vi "Change Setting.vi"(7 "Data":string, 8 "error in (no error)":errorcluster, 9 "Device and Axis":string, 10 "Setting":string, 11 "VISA resource name":refnum<visa-resource-name>) -> (0 "error out":errorcluster, 3 "VISA resource name out":refnum<visa-resource-name>)   [LabVIEW 2013, in "Zaber A Series.lvlib"]
doc: "Changes a setting from the device. Omitting the Device and Axis will change the settings of all connected devices. See a list of settings available here: http://www.zaber.com/wiki/Manuals/ASCII_Protocol_Manual#Device_Settings. You do not need to include the 'set' command with this VI, you only need to input the setting you'd like to change. \n\nThe Detect Devices VI is designed to provide an easy list of valid Device and Axis inputs. \n\nThis VI requires that the Initialize VI has been called with the same serial port."
uses:
  Zaber A Series.lvlib
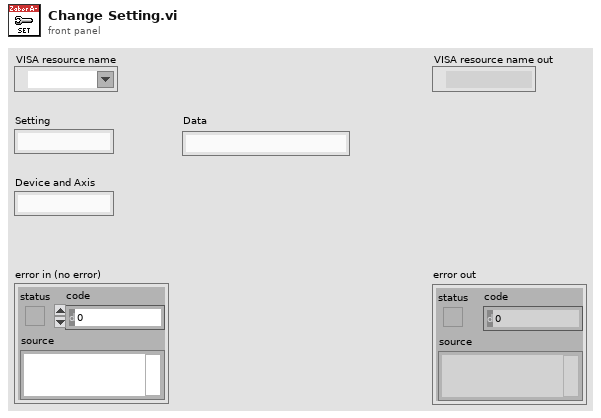
[diagram p1: front panel]
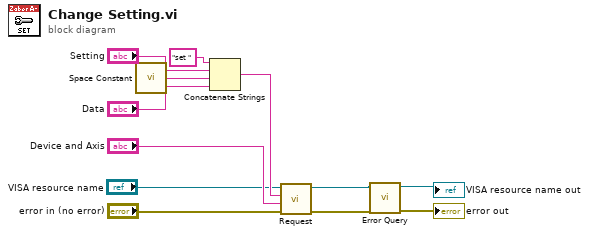
[diagram p0: block diagram]
diagram:
  n1 = call <vilib>:"Space Constant.vi"() -> ("String"=w10:string)
  n2 = Concatenate Strings("set " ("string"), "Setting", w10, "Data") -> (w8:string)
  n3 = call "Request.vi"("error in (no error)"="error in (no error)", "Device and Axis"="Device and Axis", "Command String"=w8, "VISA resource name"="VISA resource name") -> ("error out"=w2:errorcluster, "VISA resource name out"=w4:refnum<visa-resource-name>)  [unwired: 3 in, 3 out]
  n4 = call "Error Query.vi"("error in (no error)"=w2, "VISA resource name"=w4) -> ("error out"=→"error out":errorcluster, "VISA resource name out"=→"VISA resource name out":refnum<visa-resource-name>)  [unwired: 6 in, 2 out]
